vi "数据传输配置表.vi"() -> ()   [LabVIEW 2016, in "数据传输系统.lvlib"]
panel:
  in  "枚举":T1(ring)
  in  "参数数值":T2={"CODMn"=TRUE, "CODCr"=TRUE, "DO"=TRUE, "铜"=TRUE, "PH"=TRUE, "氨氮"=TRUE, "比电导率"=TRUE, "水温"=TRUE, "COD"=TRUE, "浊度"=TRUE, "总氮"=TRUE, "总磷"=TRUE, "叶绿素a"=TRUE, "藻密度"=TRUE, "水位"=TRUE, "流速"=TRUE, "瞬时流量"=TRUE, "累积流量"=TRUE, "亚硝酸盐"=TRUE, "硫化物"=TRUE, "ORP"=TRUE, "铅"=TRUE, "ïÓ"=TRUE, "锌"=TRUE, "镍"=TRUE, "锰"=TRUE, "汞"=TRUE}
  # "单位配置系数"
  # "上传功能码ST"
  # "小时数据上传触发方式"
  # "因子编码"
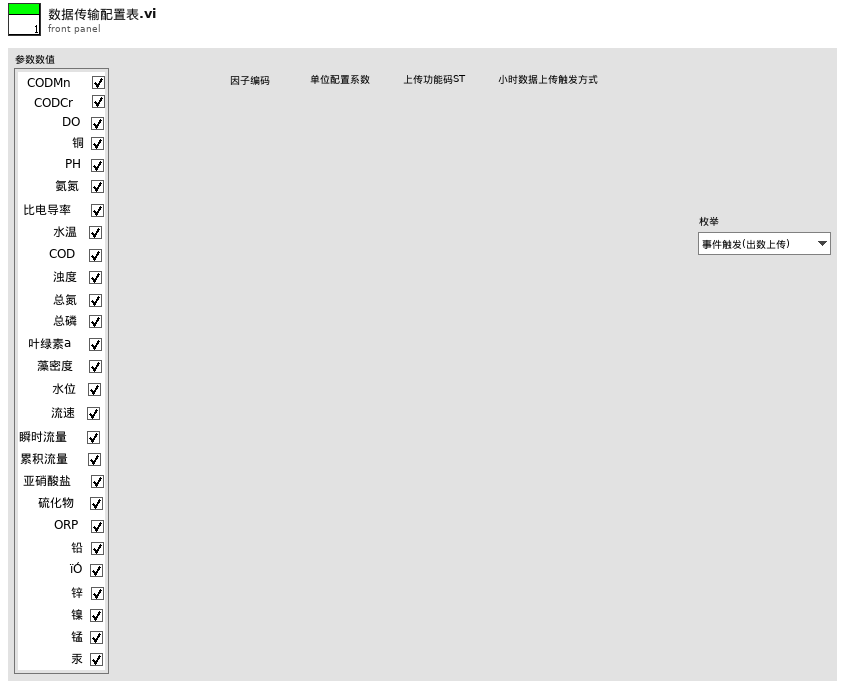
[diagram p1: front panel]
types:
  T1 = enum16{"事件触发(出数上传)", "等时间间隔10分钟", "等时间间隔20分钟", "等时间间隔30分钟", "整点上传"}
  T2 = cluster{"CODMn":bool, "CODCr":bool, "DO":bool, "铜":bool, "PH":bool, "氨氮":bool, "比电导率":bool, "水温":bool, "COD":bool, "浊度":bool, "总氮":bool, "总磷":bool, "叶绿素a":bool, "藻密度":bool, "水位":bool, "流速":bool, "瞬时流量":bool, "累积流量":bool, "亚硝酸盐":bool, "硫化物":bool, "ORP":bool, "铅":bool, "ïÓ":bool, "锌":bool, "镍":bool, "锰":bool, "汞":bool}
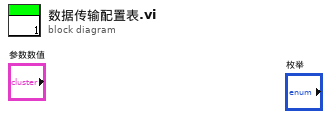
[diagram p0: block diagram]
diagram:
